vi "EXO存单表数据.vi"(0 "data":T1={"时间"=timestamp(0 s since 1904-01-01), "测量模式"="水样测试", "数据类型"="N", "数据标识"="N", "湖面水深"=0.0, "缆绳下放长度"=0.0, "层数"=0, "row"=0, "水温"=0.0, "比电导率"=0.0, "电导率"=0.0, "盐度"=0.0, "总溶解固体"=0.0, "pH"=0.0, "pHmV"=0.0, "ORP"=0.0, "饱和度"=0.0, "DO"=0.0, "浊度"=0.0, "叶绿素a"=0.0, "蓝绿藻"=0.0, "水深"=0.0, "设置水深"=0.0}) -> ()   [LabVIEW 2016, in "main.lvlib"]
uses:
  main.lvlib
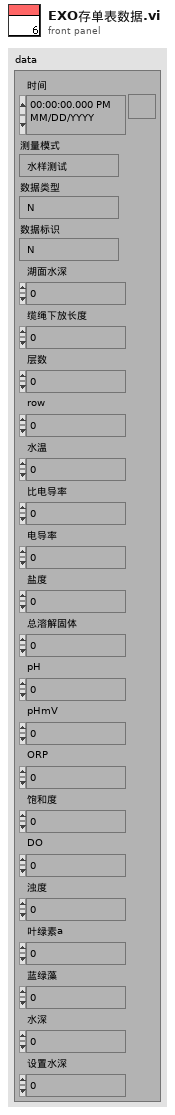
[diagram p1: front panel]
types:
  T1 = typedef "剖面数据_EXO2.ctl" = cluster{"时间":timestamp, "测量模式":string, "数据类型":string, "数据标识":string, "湖面水深":sgl, "缆绳下放长度":sgl, "层数":u16, "row":u16, "水温":sgl, "比电导率":sgl, "电导率":sgl, "盐度":sgl, "总溶解固体":sgl, "pH":sgl, "pHmV":sgl, "ORP":sgl, "饱和度":sgl, "DO":sgl, "浊度":sgl, "叶绿素a":sgl, "蓝绿藻":sgl, "水深":sgl, "设置水深":sgl}
  T2 = typedef "集成多参数单参数字段定义.ctl" = cluster{"时间":timestamp, "测量模式":string, "数据类型":string, "检测值":sgl, "单位":string, "数据标识":string, "信号值":sgl, "标样参考值":sgl, "因子编码":string, "探头温度":sgl, "LastTime":timestamp}
  T3 = typedef "checkbox.ctl" = bool
  T4 = cluster{"水温":T3, "电导率":T3, "pH":T3, "ORP":T3, "DO":T3, "浊度":T3, "叶绿素a":T3, "蓝绿藻":T3, "盐度":T3}
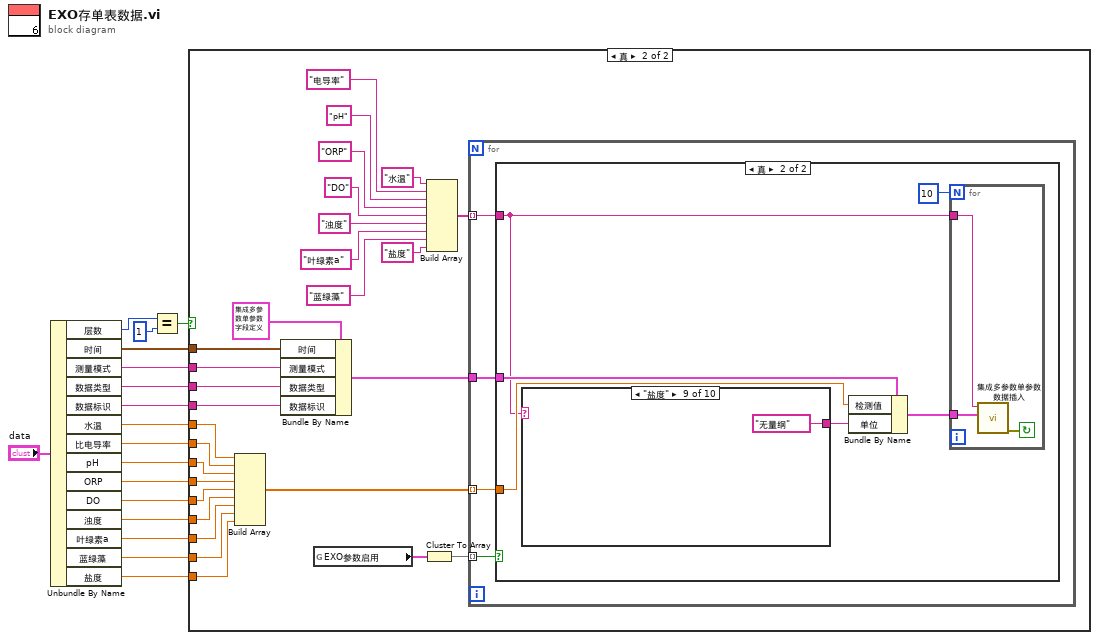
[diagram p0: block diagram]
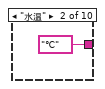
[diagram p5: hidden frame]
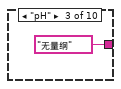
[diagram p6: hidden frame]
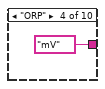
[diagram p7: hidden frame]
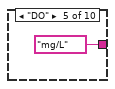
[diagram p8: hidden frame]
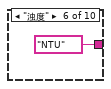
[diagram p9: hidden frame]
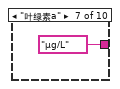
[diagram p10: hidden frame]
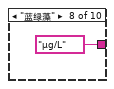
[diagram p11: hidden frame]
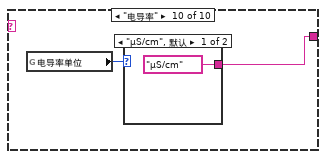
[diagram p12: hidden frame]
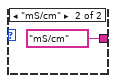
[diagram p13: hidden frame]
diagram:
  n1 = Unbundle By Name("data") -> ("层数"=w5:u16, "时间"=w16:timestamp, "测量模式"=w15:string, "数据类型"=w14:string, "数据标识"=w13:string, "水温"=w12:sgl, "比电导率"=w11:sgl, "pH"=w10:sgl, "ORP"=w9:sgl, "DO"=w8:sgl, "浊度"=w7:sgl, "叶绿素a"=w6:sgl, "蓝绿藻"=w2:sgl, "盐度"=w1:sgl)
  n2 = Equal?(x=w5, y=u16 1) -> (x = y?=w3:bool)
  n3 = case shown="真" w3 {
    tunnel: w16 -> [_ w44]
    tunnel: w15 -> [_ w43]
    tunnel: w14 -> [_ w42]
    tunnel: w13 -> [_ w41]
    tunnel: w12 -> [_ w40]
    tunnel: w11 -> [_ w39]
    tunnel: w10 -> [_ w38]
    tunnel: w9 -> [_ w37]
    tunnel: w8 -> [_ w36]
    tunnel: w7 -> [_ w35]
    tunnel: w6 -> [_ w34]
    tunnel: w2 -> [_ w19]
    tunnel: w1 -> [_ w18]
    frame False {
    }
    frame True {
      n4 = Build Array(w40, w39, w38, w37, w36, w35, w34, w19, w18) -> (w24:sgl[])
      n5 = Bundle By Name(cluster=T2 {"时间"=timestamp(0 s since 1904-01-01), "测量模式"="水样测试", "数据类型"="N", "检测值"=0.0, "单位"="", "数据标识"="N", "信号值"=0.0, "标样参考值"=0.0, "因子编码"="", "探头温度"=0.0, "LastTime"=timestamp(0 s since 1904-01-01)} ("data"), "时间"=w44, "测量模式"=w43, "数据类型"=w42, "数据标识"=w41) -> (w26:T2)
      n6 = global read "全局断电保存变量.vi" "EXO参数启用"() -> (w23:T4)
      n7 = Cluster To Array(cluster=w23) -> (array=w22:T3[])
      n8 = Build Array("水温", "电导率", "pH", "ORP", "DO", "浊度", "叶绿素a", "蓝绿藻", "盐度") -> (w25:string[])
      n9 = for {
        tunnel: w26 -> [w49]
        tunnel: w25 -> [w47] mode=indexing
        tunnel: w24 -> [w48] mode=indexing
        tunnel: w22 -> [w46] mode=indexing
        n10 = case shown="真" w46 {
          tunnel: w49 -> [_ w55]
          tunnel: w48 -> [_ w54]
          tunnel: w47 -> [_ w51]
          frame False {
          }
          frame True {
            n11 = case shown="\"盐度\"" w51 {
              tunnel: [_ "℃" ("单位") "无量纲" ("单位") "mV" ("单位") "mg/L" ("单位") "NTU" ("单位") "μg/L" ("单位") "μg/L" ("单位") "无量纲" ("单位") w64] -> w50
              frame Default {
              }
              frame "水温" {
              }
              frame "pH" {
              }
              frame "ORP" {
              }
              frame "DO" {
              }
              frame "浊度" {
              }
              frame "叶绿素a" {
              }
              frame "蓝绿藻" {
              }
              frame "盐度" {
              }
              frame "电导率" {
                n12 = global read "全局断电保存变量.vi" "电导率单位"() -> (w65:enum16{"μS/cm", "mS/cm"})
                n13 = case shown="\"μS/cm\", 默认" w65 {
                  tunnel: ["μS/cm" ("单位") "mS/cm" ("单位")] -> w64
                  frame "μS/cm", Default {
                  }
                  frame "mS/cm" {
                  }
                }
              }
            }
            n14 = Bundle By Name(cluster=w55, "检测值"=w54, "单位"=w50) -> (w53:T2)
            n15 = for {
              N: 10 -> [_]
              tunnel: w51 -> [w70]
              tunnel: w53 -> [w69]
              stop <- w68 continue-if-true
              n16 = call "集成多参数单参数数据插入.vi"("Tabe Name"=w70, "data"=w69) -> ("错误输出"=w68:errorcluster)  [unwired: 8 in]
            }
          }
        }
      }
    }
  }
